vi "DSA_Display (subVI).vi"(8 "error in (no error)":errorcluster, 9 "view":cluster{"Channel":u16, "View":u16} {"View" items=["Magnitude", "Phase", "Coherence (FRF only)"]; "Channel" items=["Channel A (stimulus)", "Channel B (response)"]}, 10 "DSA settings":T1={"function"=enum."Frequency response", "baseband span"=20000.0, "window"=enum."Hanning", "resolution (# of lines)"=800}, 11 "stimulus and response":cluster{"f0":dbl, "df":dbl, "Y":dbl[]}[](array[cluster])) -> (0 "error out":errorcluster, 2 "X Units":string, 3 "selected display":cluster{"f0":dbl, "df":dbl, "Y":dbl[]})   [LabVIEW 2023]
doc: "Displays the appropriate waveform as selected in the \"View\" selector"
panel:
  in  "Time":string="Time (s)"
  in  "Frequency":string="Frequency (Hz)"
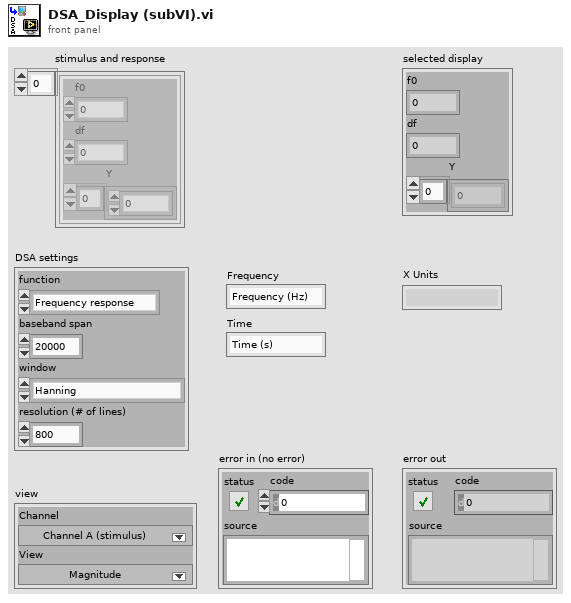
[diagram p1: front panel]
types:
  T1 = cluster{"function":enum16{"Windowed time", "Power Spectrum", "FFT (Mag-Phase)", "Cross Power spectrum", "Frequency response"}, "baseband span":dbl, "window":enum16{"None ", "Hanning", "Hamming", "Blackman-Harris", "Exact Blackman", "Blackman", "Flat Top", "4 Term B-Harris ", "7 Term B-Harris", "Low Sidelobe"}, "resolution (# of lines)":u32}
  T2 = enum16{"Windowed time", "Power Spectrum", "FFT (Mag-Phase)", "Cross Power spectrum", "Frequency response"}
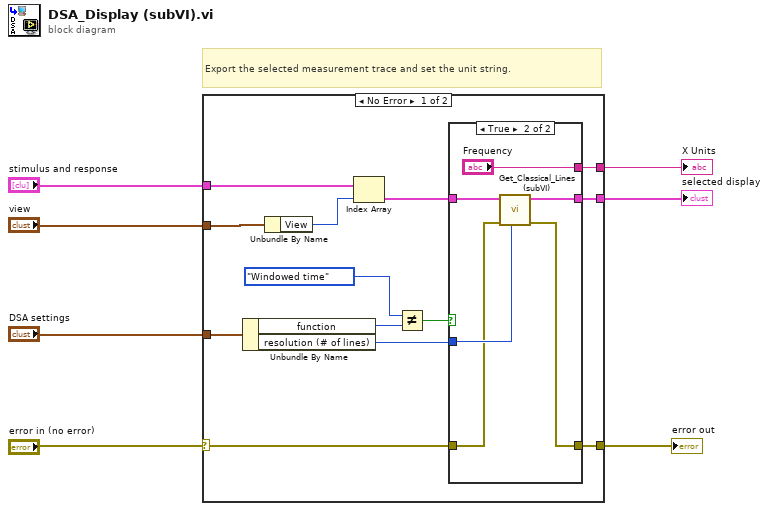
[diagram p0: block diagram]
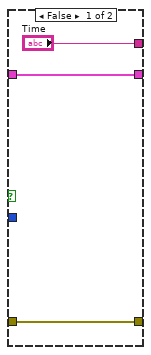
[diagram p2: hidden frame]
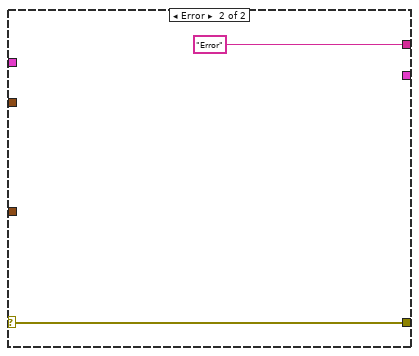
[diagram p3: hidden frame]
diagram:
  # "Export the selected measurement trace and set the unit string."
  n1 = case shown="No Error" "error in (no error)" {
    selector: "error in (no error)" -> [w11 w31]
    tunnel: "stimulus and response" -> [w20 _]
    tunnel: "view" -> [w18 _]
    tunnel: "DSA settings" -> [w17 _]
    tunnel: [w10 w31] -> w3
    tunnel: [w9 "Error" ("X Units")] -> w2
    tunnel: [w8 _] -> w1
    frame No Error {
      n2 = Unbundle By Name(w17) -> ("function"=w15:T2, "resolution (# of lines)"=w12:u32)
      n3 = Unbundle By Name(w18) -> ("View"=w19:u16)
      n4 = Index Array(array=w20, index=w19) -> (element=w13:cluster{"f0":dbl, "df":dbl, "Y":dbl[]})
      n5 = Not Equal?(x=T2."Windowed time" ("Function"), y=w15) -> (x != y?=w14:bool)
      n6 = case shown="True" w14 {
        tunnel: w13 -> [w23 w29]
        tunnel: [w23 w28] -> w8
        tunnel: ["Time" "Frequency"] -> w9
        tunnel: w12 -> [_ w26]
        tunnel: w11 -> [w21 w25]
        tunnel: [w21 w24] -> w10
        frame False {
        }
        frame True {
          n7 = call "Get_Classical_Lines (subVI).vi"("resolution (# of lines)"=w26, "error in (no error)"=w25, "power spectrum"=w29) -> ("error out"=w24:errorcluster, "spectral lines"=w28:cluster{"f0":dbl, "df":dbl, "Y":dbl[]})  [unwired: 6 in, 1 out]
        }
      }
    }
    frame Error {
    }
  }
  "error out" <- w3
  "X Units" <- w2
  "selected display" <- w1
